vi "Getunits.vi"(8 "error in (no error)":errorcluster, 11 "OneOfTemplate in":refnum<class "nidaqmx_grpc_CreateCIFreqChanRequest_units_enum.lvclass">) -> (0 "error out":errorcluster, 2 "Get_Val":T1, 3 "OneOfTemplate out":refnum<class "nidaqmx_grpc_CreateCIFreqChanRequest_units_enum.lvclass">)   [LabVIEW 2021, in "NI_DAQmx_client.lvlib" / "nidaqmx_grpc_CreateCIFreqChanRequest_units_enum.lvclass"]
uses:
  nidaqmx_grpc_CreateCIFreqChanRequest_units_enum.lvclass
  nidaqmx_grpc_FrequencyUnits3.ctl
  nidaqmx_grpc_CreateCIFreqChanRequest_units_enum.lvclass/nidaqmx_grpc_CreateCIFreqChanRequest_units_enum.ctl
  NI_DAQmx_client.lvlib
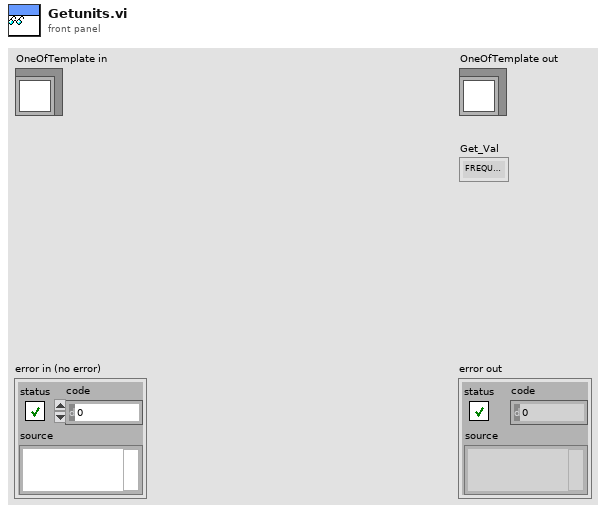
[diagram p1: front panel]
types:
  T1 = typedef "NI_DAQmx_client.lvlib/nidaqmx_grpc_FrequencyUnits3.ctl" = enum32{"FREQUENCY_UNITS3_UNSPECIFIED", "FREQUENCY_UNITS3_HZ", "FREQUENCY_UNITS3_TICKS", "FREQUENCY_UNITS3_FROM_CUSTOM_SCALE"}
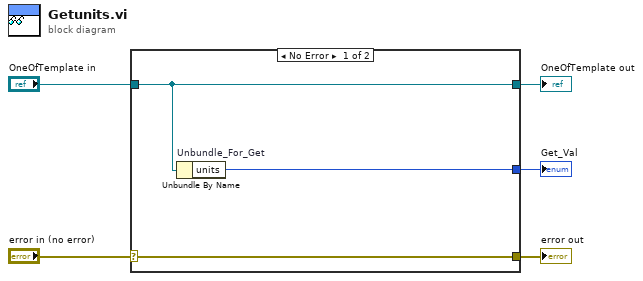
[diagram p0: block diagram]
diagram:
  n1 = case shown="No Error" "error in (no error)" {
    selector: "error in (no error)" -> [w8 w9]
    tunnel: [w8 w9] -> w4
    tunnel: [w7 w10] -> w2
    tunnel: "OneOfTemplate in" -> [w7 w10]
    tunnel: [w6 _] -> w1
    frame No Error {
      n2 = Unbundle By Name "Unbundle_For_Get"(w7) -> ("units"=w6:T1)
    }
    frame Error {
    }
  }
  "error out" <- w4
  "OneOfTemplate out" <- w2
  "Get_Val" <- w1
